vi "getAcquisitionData.vi"(6 "Delay between send and receive [ms]":i32=100, 8 "error in (no error)":errorcluster, 11 "CCD in":refnum<class "CCD.lvclass">) -> (0 "error out":errorcluster, 1 "results-JSON string":string, 2 "Aquisitions":T1[](array[typedef]), 3 "CCD out":refnum<class "CCD.lvclass">)   [LabVIEW 2023, in "horiba.lvlib" / "CCD.lvclass"]
doc: "The acquisition description string consists of the following information:\n\nacqIndex: Acquisition number\nroiIndex: Region of Interest number\nxOrigin: ROI’s X Origin\nyOrigin: ROI’s Y Origin\nxSize: ROI’s X Size\nySize: ROI’s Y Size\nxBinning: ROI’s X Bin\nyBinning: ROI’s Y Bin\nTimestamp: This is a timestamp that relates to the time when the all the programmed acquisitions have completed. The data from all programmed acquisitions are retrieved from the CCD after all acquisitions have completed, therefore the same timestamp is used for all acquisitions.\nCommand Parameters:\n\n\nReturn Results:\n\nresults description\nacquisition String. Acquisition data.\nExample command:\n\nExample response:\n\n{\n \"command\": \"ccd_getAcquisitionData\",\n \"errors\": [],\n \"id\": 1234,\n \"results\": {\n \"acquisition\": [\n {\n \"acqIndex\": 1,\n \"roi\":\n [\n {\n \"roiIndex\": 1,\n \"xBinning\": 1,\n \"xOrigin\": 1,\n \"xSize\": 8,\n \"xyData\": [\n [\n 885.6389770507812,\n 976\n ],\n [w\n 885.2899780273438,\n 975\n ],\n [\n 884.9409790039062,\n 979\n ],\n [\n 884.593017578125,\n 976\n ],\n}"
uses:
  CCD.lvclass
  acquisitionData.ctl
  CCDImageData.ctl
  20f7d3bd-08ac-4524-9bed-df36c1da25a0.vi
  <vilib>/JDP Science/JSONtext/Variant to JSON Text.vi
  <vilib>/JDP Science/JSONtext/Set Item.vi
  <vilib>/JDP Science/JSONtext/LVClass Serializer/JSONtext LVClass Serializer.lvclass
  CCD.lvclass/CCD.ctl
  GenericDevice/GenericDevice.lvclass
panel:
  # "Connector Pane"
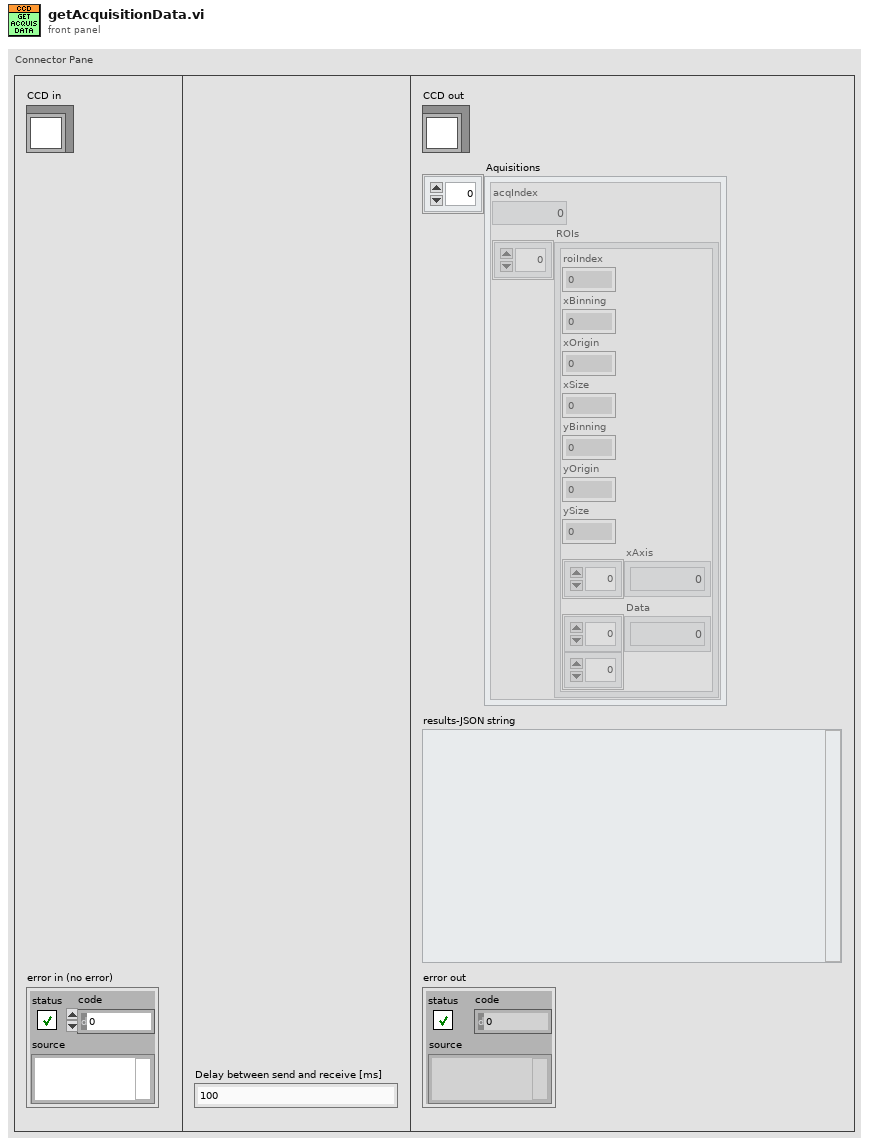
[diagram p1: front panel]
types:
  T1 = typedef "horiba.lvlib/CCD.lvclass/acquisitionData.ctl" = cluster{"acqIndex":i32, "ROIs":T2[]}
  T2 = typedef "horiba.lvlib/CCD.lvclass/CCDImageData.ctl" = cluster{"roiIndex":i32, "xBinning":i32, "xOrigin":i32, "xSize":i32, "yBinning":i32, "yOrigin":i32, "ySize":i32, "xAxis":dbl[], "Data":dbl[][]}
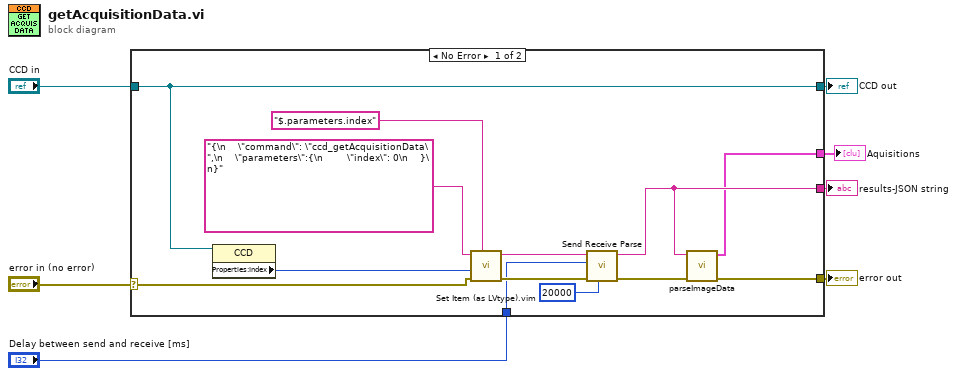
[diagram p0: block diagram]
diagram:
  n1 = case shown="No Error" "error in (no error)" {
    selector: "error in (no error)" -> [w16 w22]
    tunnel: [w10 w22] -> w6
    tunnel: [w18 w21] -> w4
    tunnel: "CCD in" -> [w18 w21]
    tunnel: "Delay between send and receive [ms]" -> [w14 _]
    tunnel: [w12 _] -> w2
    tunnel: [w9 _] -> w1
    frame No Error {
      n2 = property class="CCD"(reference=w18) -> ("Properties:Index"=w17:i32)  [unwired: 1 in, 2 out]
      n3 = call "Set Item (as LVtype).vim"("$Path or Item Name"="$.parameters.index", "error in (no error)"=w16, "Anything"=w17, "JSON"="{\n    \"command\": \"ccd_getAcquisitionData\",\n    \"parameters\":{\n        \"index\": 0\n    }\n}") -> ("error out"=w15:errorcluster, "<JSON>"=w13:string)  [unwired: 4 in, 1 out]
      n4 = call "Send Receive Parse.vi"("timeout in ms (-1)"=20000, "error in"=w15, "Delay between send and receive [ms]"=w14, "<JSON>"=w13) -> ("error out"=w11:errorcluster, "results-JSON string"=w12:string)  [unwired: 5 in, 1 out]
      n5 = call "parseImageData.vi"("error in (no error)"=w11, "results-JSON string"=w12) -> ("error out"=w10:errorcluster, "Aquisitions"=w9:T1[])  [unwired: 8 in]
    }
    frame Error {
    }
  }
  "error out" <- w6
  "CCD out" <- w4
  "results-JSON string" <- w2
  "Aquisitions" <- w1
